vi "Variant To Formatted Strings.vi"(4 "Registry Variant Accessor in":refnum<class "CConfig Variant Accessor.lvclass">, 5 "Formatting (auto)":string[](array[string]), 6 "Variant":variant, 7 "Formatting (auto)":string, 8 "error in (no error)":errorcluster, 9 "Read values? [T]":bool=TRUE, 10 "Multiply":variant, 11 "Carya Config in":refnum<class "Carya Config.lvclass">) -> (0 "error out":errorcluster, 1 "Labels":string[](array[string]), 2 "Formatted Strings":string[](array[string]), 3 "Carya Config out":refnum<class "Carya Config.lvclass">)   [LabVIEW 2013, in "Carya Config.lvclass"]
doc: "Copyright 2018, Carya Automatisering, Wiebe Walstra."
uses:
  Carya Config.lvclass
  CConfig Variant Accessor/CConfig Variant Accessor.lvclass
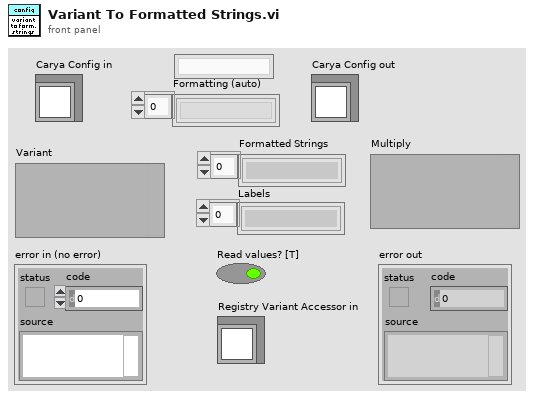
[diagram p1: front panel]
types:
  T1 = typedef "VariantType.lvlib/Type.ctl" = enum8{"Invalid Type", "Void", "I8", "I16", "I32", "I64", "U8", "U16", "U32", "U64", "Single Float", "Double Float", "Extended Float", "Single Complex", "Double Complex", "Extended Complex", "Enum U8", "Enum U16", "Enum U32", "Enum U64", "Single Float With Unit", "Double Float With Unit", "Extended Float With Unit", "Single Complex with Unit", "Double Complex with Unit", "Extended Complex with Unit", "Boolean", "String", "Path", "Picture", "Tag", "Array", "Cluster", "Variant", "LV Variant", "Waveform", "Timestamp", "Digital Waveform", "Digital Data", "ExpressData", "Refnum", "External Data", "VI", "Poly VI", "LabVIEW Class Instance", "Fixed Point"}
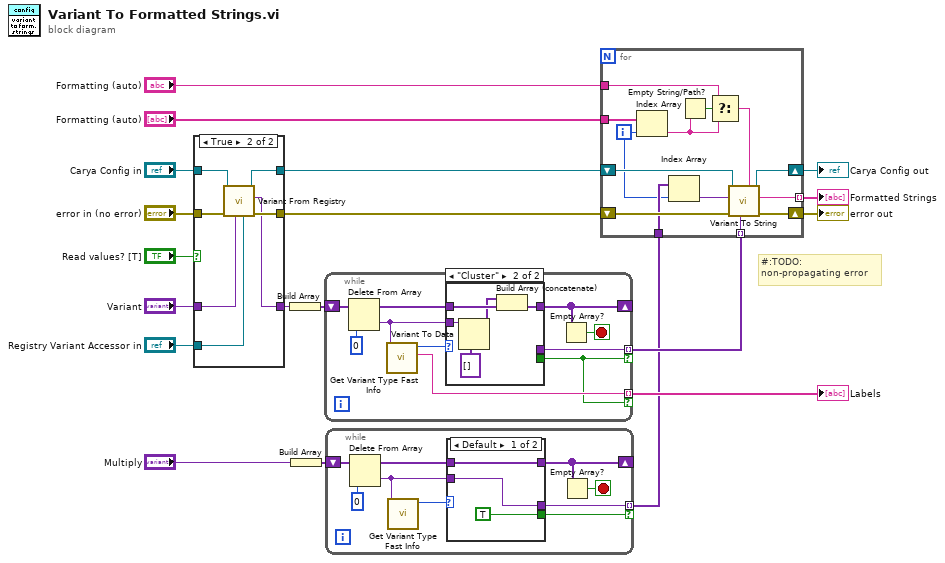
[diagram p0: block diagram]
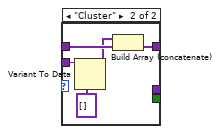
[diagram p3: hidden frame]
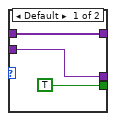
[diagram p4: hidden frame]
diagram:
  # "#:TODO:\nnon-propagating error"
  n1 = case shown="True" "Read values? [T]" {
    tunnel: "error in (no error)" -> [w21 w29]
    tunnel: [w21 w28] -> w7
    tunnel: "Carya Config in" -> [w22 w27]
    tunnel: [w22 w26] -> w5
    tunnel: "Registry Variant Accessor in" -> [_ w25]
    tunnel: "Variant" -> [w20 w24]
    tunnel: [w20 w23] -> w2
    frame False {
    }
    frame True {
      n2 = call "Variant From Registry.vi"("Registry Variant Accessor in"=w25, "Variant"=w24, "error in (no error)"=w29, "Carya Config in"=w27) -> ("error out"=w28:errorcluster, "Variant"=w23:variant, "Carya Config out"=w26:refnum<class "Carya Config.lvclass">)  [unwired: 4 in, 1 out]
    }
  }
  n3 = Build Array(w2) -> (w14:variant[])
  n4 = Build Array("Multiply") -> (w10:variant[])
  n5 = while {
    shift-right: [w34] -> _
    shift-left: w14 -> [w39]
    tunnel: [w32] -> w13 mode=indexing if=w30
    tunnel: [w31] -> w12 mode=indexing if=w30
    stop <- w33 stop-if-true
    n6 = Delete From Array(array=w39, index=0) -> (deleted portion=w35:variant, array with subset deleted=w36:variant[])  [unwired: 1 in]
    n7 = call "Get Variant Type Fast Info.vi"("Variant"=w35) -> ("Name"=w31:string, "Type Enum"=w37:T1)  [unwired: 6 in, 3 out]
    n8 = case shown="\"Cluster\"" w37 {
      tunnel: w36 -> [w42 w47]
      tunnel: [w42 w46] -> w34
      tunnel: w35 -> [w41 w45]
      tunnel: [w41 _] -> w32
      tunnel: [TRUE _] -> w30
      frame Default {
      }
      frame "Cluster" {
        n9 = Variant To Data(type=variant[] [], Variant=w45) -> (data=w43:variant[])  [unwired: 1 in, 1 out]
        n10 = Build Array (concatenate)(w43, w47) -> (w46:variant[])
      }
    }
    n11 = Empty Array?(array=w34) -> (empty?=w33:bool)
  }
  "Labels" <- w12
  n12 = while {
    shift-right: [w51] -> _
    shift-left: w10 -> [w56]
    tunnel: [w49] -> w8 mode=indexing if=w48
    stop <- w50 stop-if-true
    n13 = Delete From Array(array=w56, index=0) -> (deleted portion=w52:variant, array with subset deleted=w53:variant[])  [unwired: 1 in]
    n14 = call "Get Variant Type Fast Info.vi"("Variant"=w52) -> ("Type Enum"=w54:T1)  [unwired: 6 in, 4 out]
    n15 = case shown="Default" w54 {
      tunnel: w53 -> [w59 w64]
      tunnel: [w59 w63] -> w51
      tunnel: w52 -> [w58 w62]
      tunnel: [w58 _] -> w49
      tunnel: [TRUE _] -> w48
      frame Default {
      }
      frame "Cluster" {
        n16 = Variant To Data(type=variant[] [], Variant=w62) -> (data=w60:variant[])  [unwired: 1 in, 1 out]
        n17 = Build Array (concatenate)(w60, w64) -> (w63:variant[])
      }
    }
    n18 = Empty Array?(array=w51) -> (empty?=w50:bool)
  }
  n19 = for {
    tunnel: w13 -> [w76] mode=indexing
    tunnel: "Formatting (auto)" -> [w74]
    tunnel: [w75] -> w15 mode=indexing
    shift-right: [w72] -> w18
    shift-left: w7 -> [w77]
    shift-right: [w73] -> w19
    shift-left: w5 -> [w78]
    tunnel: "Formatting (auto)" -> [w68]
    tunnel: w8 -> [w67]
    i -> [w66]
    n20 = Index Array(array=w74, index=w66) -> (element=w70:string)
    n21 = Index Array(array=w67, index=w66) -> (element=w65:variant)
    n22 = Empty String/Path?(string/path=w70) -> (empty?=w71:bool)
    n23 = Select(t=w68, s=w71, f=w70) -> (s? t:f=w69:string)
    n24 = call-dynamic "Variant To String.vi"("Formatting (auto)"=w69, "Variant Type\\default"=w76, "error in (no error)"=w77, "Multiply"=w65, "Registry Object"=w78) -> ("error out"=w72:errorcluster, "String"=w75:string, "Registry Object"=w73:refnum<class "Carya Config.lvclass">)  [unwired: 4 in]
  }
  "error out" <- w18
  "Carya Config out" <- w19
  "Formatted Strings" <- w15
